vi "Select Datatype.vi"(10 "data":string[][](array[string]), 11 "Devicetype":string[](array[string])) -> (3 "Datatype":string[](array[string]))   [LabVIEW 2013]
panel:
  out "size(s)":i32
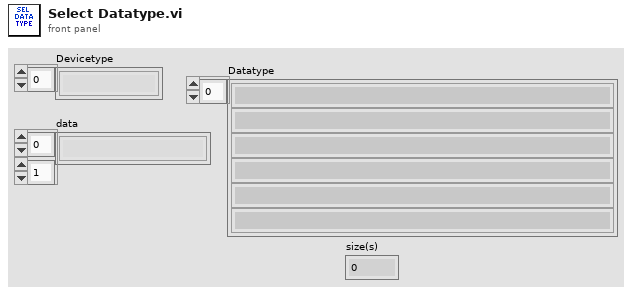
[diagram p1: front panel]
types:
  T1 = typedef "mysql_authentication.ctl" = cluster{"User":string, "Password":string, "Database":string}
  T2 = cluster{"Port":u16, "IP Address":string, "Authentication":T1}
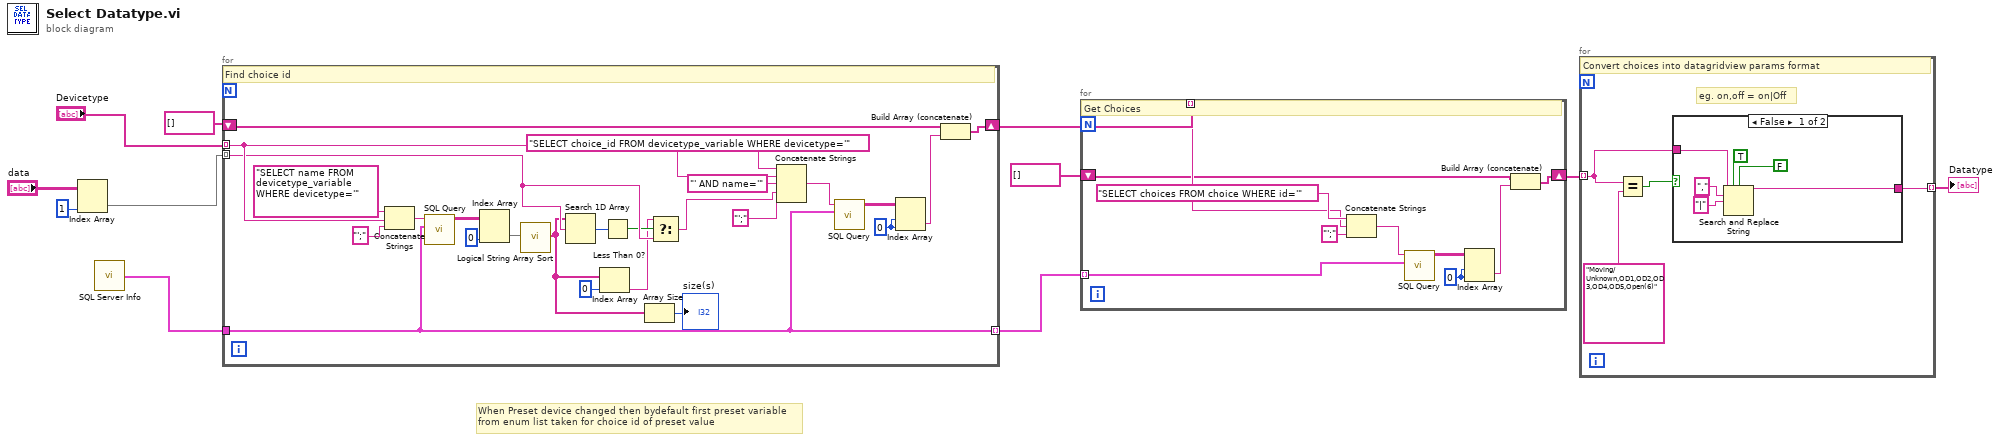
[diagram p0: block diagram]
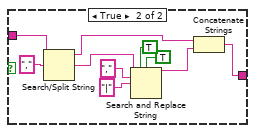
[diagram p2: hidden frame]
diagram:
  # "When Preset device changed then bydefault first preset variable\nfrom enum list taken for choice id of preset value"
  n1 = Index Array(array="data", index (col)=1 ("disabled index (col)")) -> (element=w6:string[])  [unwired: 1 in]
  n2 = call "SQL Server Info.vi"() -> ("SQL Server Info"=w1:T2)
  n3 = for {
    shift-right: [w30] -> w8
    shift-left: string[] [] -> [w32]
    tunnel: "Devicetype" -> [w27] mode=indexing
    tunnel: w1 -> [w24]
    tunnel: w6 -> [w26] mode=indexing
    tunnel: [w24] -> w9 mode=indexing
    w33 = 0 ("disabled index (col)")
    # "Find choice id"
    n4 = Concatenate Strings("SELECT name FROM devicetype_variable WHERE devicetype='", w27, "';" ("string")) -> (w23:string)
    n5 = call "SQL Query.vi"("SQL Server Info"=w24, "Query"=w23) -> ("data"=w19:string[][])  [unwired: 8 in, 1 out]
    n6 = Index Array(array=w19, index (col)=0 ("disabled index (col)")) -> (element=w20:string[])  [unwired: 1 in]
    n7 = call "Logical String Array Sort.vi"("Unsorted List"=w20) -> ("Sorted List"=w13:string[])  [unwired: 18 in]
    n8 = Search 1D Array(1D array=w13, element=w26) -> (index of element=w17:i32)  [unwired: 1 in]
    n9 = Index Array(array=w13, index=0) -> (element=w14:string)
    n10 = Less Than 0?(x=w17) -> (x < 0?=w16:bool)
    n11 = Array Size(array=w13) -> (size(s)=→"size(s)":i32)
    n12 = Select(t=w14, s=w16, f=w26) -> (s? t:f=w25:string)
    n13 = Concatenate Strings("SELECT choice_id FROM devicetype_variable WHERE devicetype='", w27, "' AND name='" ("string"), w25, "';" ("string")) -> (w35:string)
    n14 = call "SQL Query.vi"("SQL Server Info"=w24, "Query"=w35) -> ("data"=w34:string[][])  [unwired: 8 in, 1 out]
    n15 = Index Array(array=w34, index (row)=w33, index (col)=w33) -> (element=w31:string)
    n16 = Build Array (concatenate)(w32, w31) -> (w30:string[])
  }
  n17 = for {
    tunnel: w8 -> [w41] mode=indexing
    shift-right: [w38] -> w10
    shift-left: string[] [] -> [w40]
    tunnel: w9 -> [w37] mode=indexing
    w42 = 0 ("disabled index (col)")
    # "Get Choices"
    n18 = Concatenate Strings("SELECT choices FROM choice WHERE id='", w41, "';" ("string")) -> (w44:string)
    n19 = call "SQL Query.vi"("SQL Server Info"=w37, "Query"=w44) -> ("data"=w43:string[][])  [unwired: 8 in, 1 out]
    n20 = Index Array(array=w43, index (row)=w42, index (col)=w42) -> (element=w39:string)
    n21 = Build Array (concatenate)(w40, w39) -> (w38:string[])
  }
  n22 = for {
    tunnel: w10 -> [w47] mode=indexing
    tunnel: [w50] -> w11 mode=indexing
    # "eg. on,off = on|Off"
    # "Convert choices into datagridview params format"
    n23 = Equal?(x=w47, y="Moving/Unknown,OD1,OD2,OD3,OD4,OD5,Open(6)") -> (x = y?=w48:bool)
    n24 = case shown="False" w48 {
      tunnel: [w52 w58] -> w50
      tunnel: w47 -> [w51 w62]
      frame False {
        n25 = Search and Replace String(replace all?=TRUE ("replace all? (F)"), case sensitive?=FALSE ("ignore case? (F)"), input string=w51, search string=",", replace string="|" ("replace string (\"\")")) -> (result string=w52:string)  [unwired: 3 in, 3 out]
      }
      frame True {
        n26 = Search/Split String(string=w62, search string/char (-)=",") -> (substring before match=w57:string, match + rest of string=w60:string)  [unwired: 1 in, 1 out]
        n27 = Search and Replace String(replace all?=TRUE ("replace all? (F)"), case sensitive?=TRUE ("ignore case? (F)"), input string=w60, search string=",", replace string="|" ("replace string (\"\")")) -> (result string=w59:string)  [unwired: 3 in, 3 out]
        n28 = Concatenate Strings(w57, w59) -> (w58:string)
      }
    }
  }
  "Datatype" <- w11
